vi "Read.vi"(8 "error in (no error)":errorcluster, 11 "DIO Ref In":T1) -> (0 "error out":errorcluster, 2 "Values":bool[](array[boolean]), 3 "DIO Ref Out":T1)   [LabVIEW 2021, in "DIO.lvlib"]
doc: "Reads the logic levels of one or more digital I/O channels."
uses:
  <vilib>/myRIO/Instrument Drivers/Onboard IO/DIO/DIO.lvlib
  <vilib>/myRIO/Instrument Drivers/Onboard IO/DIO/typedefs/DIO Reference.ctl
  <vilib>/myRIO/Common/Instrument Driver Framework/Utilities/typedefs/myRIO Generic Hardware Reference.ctl
  <vilib>/myRIO/Common/Instrument Driver Framework/Utilities/typedefs/Hardware Version Enum.ctl
  <vilib>/myRIO/Common/Instrument Driver Framework/Utilities/typedefs/myRIO v1.0 Reference.ctl
  <vilib>/myRIO/Common/Instrument Driver Framework/Utilities/typedefs/Generic FPGA Reference.ctl
  <vilib>/myRIO/Common/Instrument Driver Framework/myRIO v1.0/DIO/typedefs/DIO Channels List.ctl
  <vilib>/myRIO/Common/Instrument Driver Framework/myRIO v1.0/DIO/typedefs/DIO Channels Enum.ctl
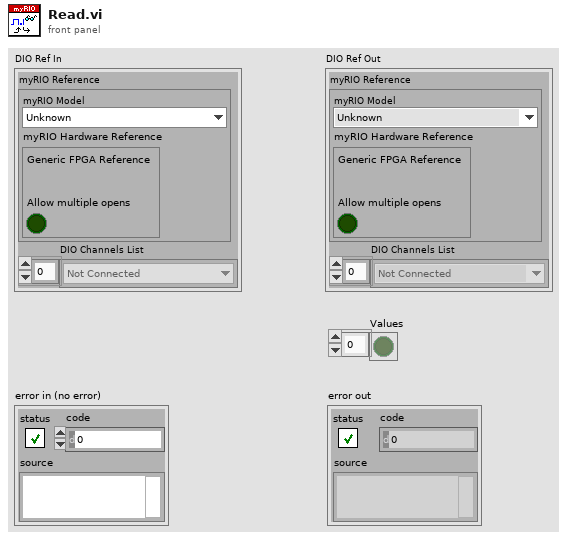
[diagram p1: front panel]
types:
  T1 = typedef "DIO.lvlib/DIO Reference.ctl" = cluster{"myRIO Reference":T2, "DIO Channels List":T6}
  T2 = typedef "myRIO Generic Hardware Reference.ctl" = cluster{"myRIO Model":T3, "myRIO Hardware Reference":T4}
  T3 = typedef "Hardware Version Enum.ctl" = enum16{"Unknown", "myRIO-1900", "myRIO-1950", "roboRIO", "NI ELVIS RIO CM", "ELVIS III"}
  T4 = typedef "myRIO v1.0 Reference.ctl" = cluster{"Generic FPGA Reference":T5, "Allow multiple opens":bool}
  T5 = typedef "Generic FPGA Reference.ctl" = refnum<k20>
  T6 = typedef "DIO Channels List.ctl" = T7[]
  T7 = typedef "DIO Channels Enum.ctl" = enum16{"Not Connected", "C/DIO0", "C/DIO1", "C/DIO2", "C/DIO3", "C/DIO4", "C/DIO5", "C/DIO6", "C/DIO7", "A/DIO0", "A/DIO1", "A/DIO2", "A/DIO3", "A/DIO4", "A/DIO5", "A/DIO6", "A/DIO7", "A/DIO8", "A/DIO9", "A/DIO10", "A/DIO11", "A/DIO12", "A/DIO13", "A/DIO14", "A/DIO15", "A/DIO16", "A/DIO17", "A/DIO18", "A/DIO19", "B/DIO0", "B/DIO1", "B/DIO2", "B/DIO3", "B/DIO4", "B/DIO5", "B/DIO6", "B/DIO7", "B/DIO8", "B/DIO9", "B/DIO10", "B/DIO11", "B/DIO12", "B/DIO13", "B/DIO14", "B/DIO15", "B/DIO16", "B/DIO17", "B/DIO18", "B/DIO19", "LED0", "LED1", "LED2", "LED3", "Button0", "DIO/DIO0", "DIO/DIO1", "DIO/DIO2", "DIO/DIO3", "DIO/DIO4", "DIO/DIO5", "DIO/DIO6", "DIO/DIO7", "DIO/DIO8", "DIO/DIO9", "SPI/CS0", "SPI/CS1", "SPI/CS2", "SPI/CS3", "LED RADIO (Green)", "LED RADIO (Red)", "LED COMM (Green)", "LED COMM (Red)", "LED MODE (Green)", "LED MODE (Red)"}
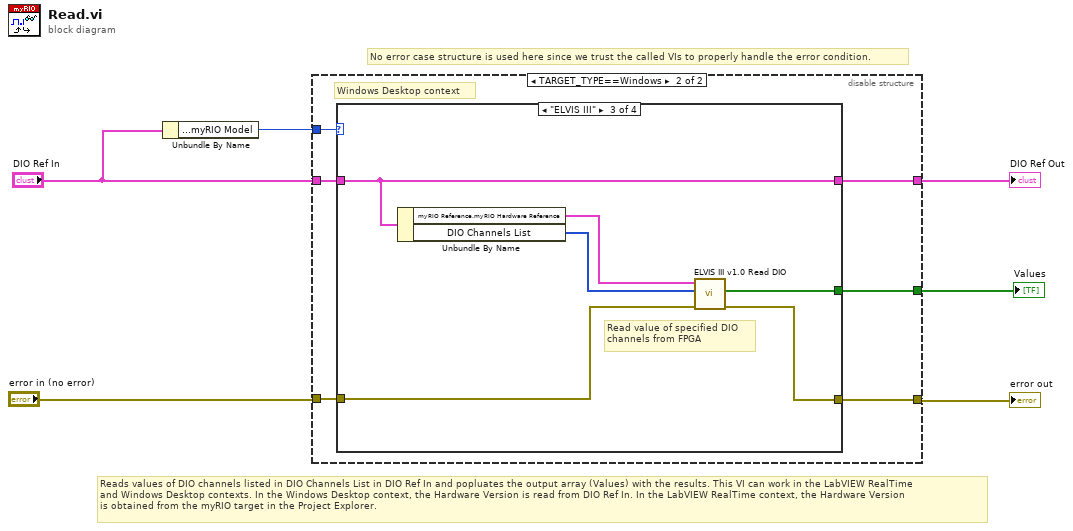
[diagram p0: block diagram]
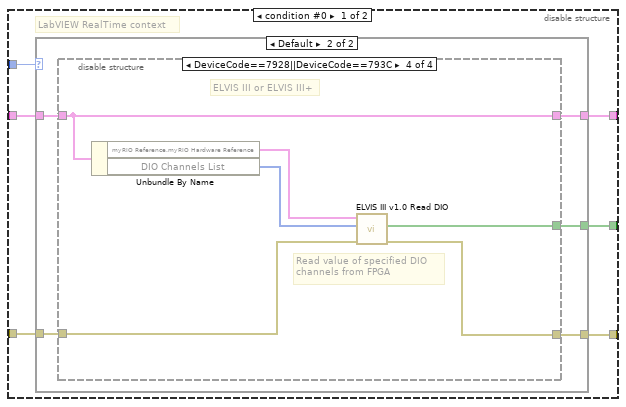
[diagram p2: hidden frame]
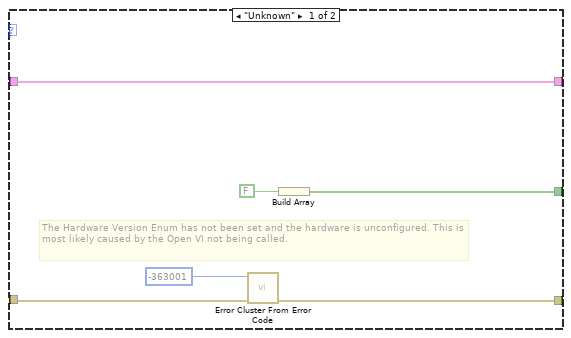
[diagram p3: hidden frame]
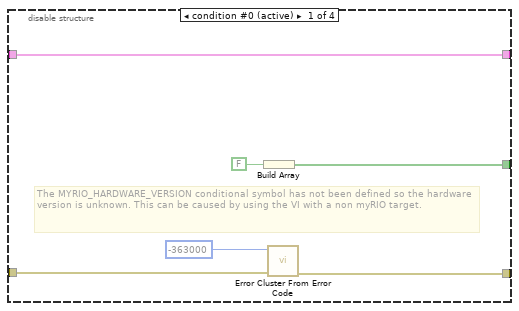
[diagram p4: hidden frame]
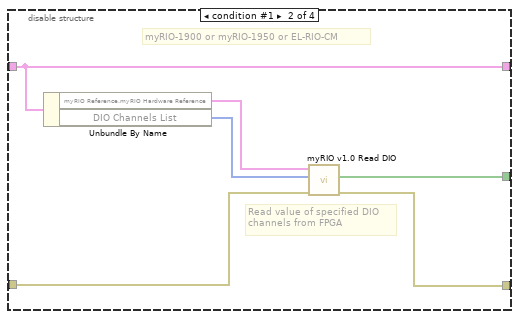
[diagram p5: hidden frame]
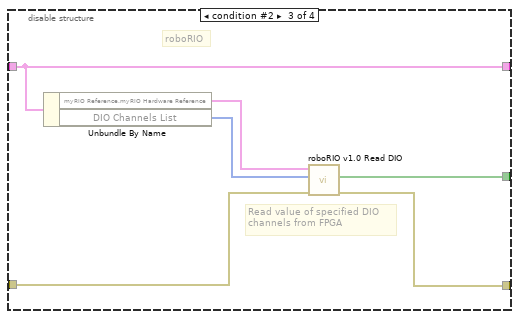
[diagram p6: hidden frame]
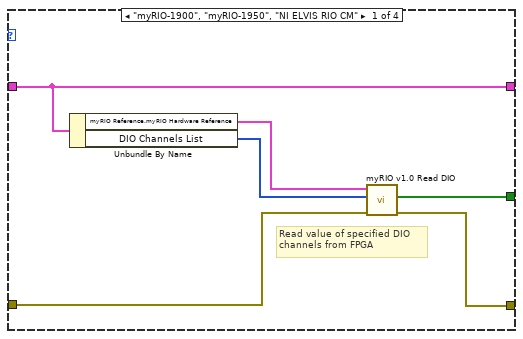
[diagram p7: hidden frame]
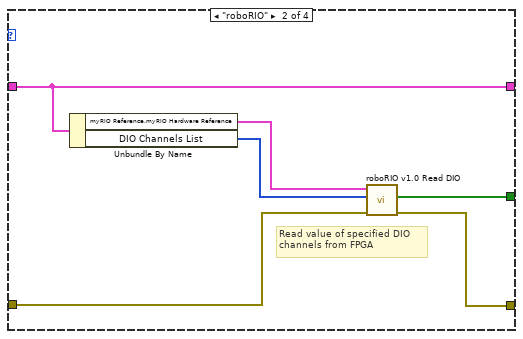
[diagram p8: hidden frame]
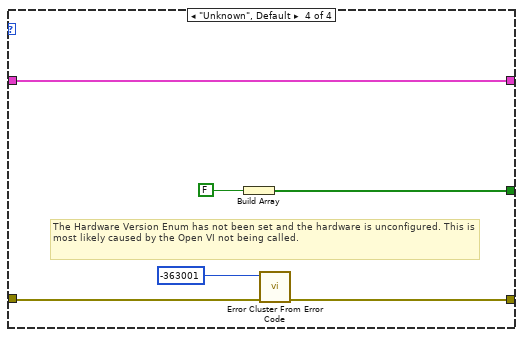
[diagram p9: hidden frame]
diagram:
  # "No error case structure is used here since we trust the called VIs to properly handle the error condition."
  # "Reads values of DIO channels listed in DIO Channels List in DIO Ref In and popluates the output array (Values) with the results. This VI can work in the LabVIEW RealTime \nand Windows Desktop contexts. In the Windows Desktop context, the Hardware Version is read from DIO Ref In. In the LabVIEW RealTime context, the Hardware Version\nis obtained from the myRIO target in the Project Explorer."
  n1 = Unbundle By Name("DIO Ref In") -> ("myRIO Reference.myRIO Model"=w1:T3)
  n2 = disable-structure shown="TARGET_TYPE==Windows" {
    disable-tunnel: [w12 w53] -> w3
    disable-tunnel: "DIO Ref In" -> [w11 w50]
    disable-tunnel: "error in (no error)" -> [w10 w52]
    disable-tunnel: [w9 w51] -> w4
    disable-tunnel: [w8 w49] -> w2
    disable-tunnel: w1 -> [w7 w48]
    frame condition #0 {
      # "LabVIEW RealTime context"
      n3 = case shown="Default" w7 {
        tunnel: [w16 w23] -> w12
        tunnel: w11 -> [w14 w22]
        tunnel: w10 -> [w17 w21]
        tunnel: [w14 w20] -> w9
        tunnel: [w15 w19] -> w8
        frame "Unknown" {
          # "The Hardware Version Enum has not been set and the hardware is unconfigured. This is most likely caused by the Open VI not being called."
          n4 = call <vilib>:"Error Cluster From Error Code.vi"("error in (no error)"=w17, "error code (0)"=-363001) -> ("error out"=w16:errorcluster)  [unwired: 7 in]
          n5 = Build Array(FALSE) -> (w15:bool[])
        }
        frame Default {
          n6 = disable-structure shown="DeviceCode==7928||DeviceCode==793C" {
            disable-tunnel: w22 -> [w26 w34 w40 w42]
            disable-tunnel: [w29 w30 w36 w44] -> w23
            disable-tunnel: [w25 w31 w37 w43] -> w19
            disable-tunnel: w21 -> [w27 w33 w39 w45]
            disable-tunnel: [w26 w34 w40 w42] -> w20
            frame condition #0 (active) {
              # "The MYRIO_HARDWARE_VERSION conditional symbol has not been defined so the hardware version is unknown. This can be caused by using the VI with a non myRIO target."
              n7 = Build Array(FALSE) -> (w25:bool[])
              n8 = call <vilib>:"Error Cluster From Error Code.vi"("error in (no error)"=w27, "error code (0)"=-363000) -> ("error out"=w29:errorcluster)  [unwired: 7 in]
            }
            frame condition #1 {
              # "myRIO-1900 or myRIO-1950 or EL-RIO-CM"
              # "Read value of specified DIO \nchannels from FPGA"
              n9 = Unbundle By Name(w34) -> ("myRIO Reference.myRIO Hardware Reference"=w35:T4, "DIO Channels List"=w32:T6)
              n10 = call <vilib>:"myRIO v1.0 Read DIO.vi"("error in (no error)"=w33, "Channel List"=w32, "myRIO Ref In"=w35) -> ("error out"=w30:errorcluster, "bool Value List"=w31:bool[])  [unwired: 6 in, 1 out]
            }
            frame condition #2 {
              # "roboRIO"
              # "Read value of specified DIO \nchannels from FPGA"
              n11 = Unbundle By Name(w40) -> ("myRIO Reference.myRIO Hardware Reference"=w41:T4, "DIO Channels List"=w38:T6)
              n12 = call <vilib>:"roboRIO v1.0 Read DIO.vi"("error in (no error)"=w39, "Channel List"=w38, "myRIO Ref In"=w41) -> ("error out"=w36:errorcluster, "bool Value List"=w37:bool[])  [unwired: 6 in, 1 out]
            }
            frame condition #3 {
              # "ELVIS III or ELVIS III+"
              # "Read value of specified DIO \nchannels from FPGA"
              n13 = Unbundle By Name(w42) -> ("myRIO Reference.myRIO Hardware Reference"=w47:T4, "DIO Channels List"=w46:T6)
              n14 = call <vilib>:"ELVIS III v1.0 Read DIO.vi"("error in (no error)"=w45, "Channel List"=w46, "myRIO Ref In"=w47) -> ("error out"=w44:errorcluster, "bool Value List"=w43:bool[])  [unwired: 6 in, 1 out]
            }
          }
        }
      }
    }
    frame condition #1 (active) {
      # "Windows Desktop context"
      n15 = case shown="\"ELVIS III\"" w48 {
        tunnel: [w55 w61 w67 w77] -> w53
        tunnel: w50 -> [w59 w65 w69 w74]
        tunnel: w52 -> [w56 w62 w66 w75]
        tunnel: [w59 w65 w69 w74] -> w51
        tunnel: [w54 w60 w68 w73] -> w49
        frame "myRIO-1900", "myRIO-1950", "NI ELVIS RIO CM" {
          # "Read value of specified DIO \nchannels from FPGA"
          n16 = Unbundle By Name(w59) -> ("myRIO Reference.myRIO Hardware Reference"=w58:T4, "DIO Channels List"=w57:T6)
          n17 = call <vilib>:"myRIO v1.0 Read DIO.vi"("error in (no error)"=w56, "Channel List"=w57, "myRIO Ref In"=w58) -> ("error out"=w55:errorcluster, "bool Value List"=w54:bool[])  [unwired: 6 in, 1 out]
        }
        frame "roboRIO" {
          # "Read value of specified DIO \nchannels from FPGA"
          n18 = Unbundle By Name(w65) -> ("myRIO Reference.myRIO Hardware Reference"=w64:T4, "DIO Channels List"=w63:T6)
          n19 = call <vilib>:"roboRIO v1.0 Read DIO.vi"("error in (no error)"=w62, "Channel List"=w63, "myRIO Ref In"=w64) -> ("error out"=w61:errorcluster, "bool Value List"=w60:bool[])  [unwired: 6 in, 1 out]
        }
        frame "ELVIS III" {
          # "Read value of specified DIO \nchannels from FPGA"
          n20 = Unbundle By Name(w69) -> ("myRIO Reference.myRIO Hardware Reference"=w71:T4, "DIO Channels List"=w70:T6)
          n21 = call <vilib>:"ELVIS III v1.0 Read DIO.vi"("error in (no error)"=w66, "Channel List"=w70, "myRIO Ref In"=w71) -> ("error out"=w67:errorcluster, "bool Value List"=w68:bool[])  [unwired: 6 in, 1 out]
        }
        frame "Unknown", Default {
          # "The Hardware Version Enum has not been set and the hardware is unconfigured. This is most likely caused by the Open VI not being called."
          n22 = Build Array(FALSE) -> (w73:bool[])
          n23 = call <vilib>:"Error Cluster From Error Code.vi"("error in (no error)"=w75, "error code (0)"=-363001) -> ("error out"=w77:errorcluster)  [unwired: 7 in]
        }
      }
    }
  }
  "DIO Ref Out" <- w4
  "error out" <- w3
  "Values" <- w2
